vi "SEN_Loop.vi"() -> ()   [LabVIEW 2023, in "Swerve_Odometry_SEN.lvlib"]
uses:
  Swerve_Odometry_SEN.lvlib
  RoboRIO Utilities/Global_STOP.vi
  ENUM_SEN_Action.ctl
  ENUM_SEN_State.ctl
  Global_SEN_Data Out.vi
  Global_CMD_SEN_Data In.vi
  Cluster_TRANSLATION2D.ctl
  Cluster_ROTATION2D.ctl
  Cluster_POSE2D.ctl
  Cluster_SWERVE_DRIVE_MODULE_POSITION.ctl
  Cluster_SWERVE_DRIVE_ODOMETRY.ctl
  SwerveDrive/Global_ACT_Data Out.vi
  PigeonIMU/Global_SEN_Data Out.vi
panel:
  out "SWERVE_DRIVE_ODOMETRY":T1={"POSE"={"TRANSLATION"={"X"=0.0, "Y"=0.0}, "ROTATION"={"VALUE"=0.0, "COS"=1.0, "SIN"=0.0}}, "GyroOffset"={"VALUE"=0.0, "COS"=1.0, "SIN"=0.0}, "PreviousAngle"={"VALUE"=0.0, "COS"=1.0, "SIN"=0.0}, "PrevTime"=0.0, "PrevModulePosition"=[], "NumModules"=0} {"PrevModulePosition"."Angle"."SIN" format="%13.4f"; "PrevModulePosition"."Angle"."COS" format="%13.4f"; "PrevModulePosition"."Angle"."VALUE" format="%13.4f"; "PreviousAngle"."SIN" format="%13.4f"; "PreviousAngle"."COS" format="%13.4f"; "PreviousAngle"."VALUE" format="%13.4f"; "GyroOffset"."SIN" format="%13.4f"; "GyroOffset"."COS" format="%13.4f"; "GyroOffset"."VALUE" format="%13.4f"; "POSE"."ROTATION"."SIN" format="%13.4f"; "POSE"."ROTATION"."COS" format="%13.4f"; "POSE"."ROTATION"."VALUE" format="%13.4f"; "POSE"."TRANSLATION"."Y" format="%14.3f"; "POSE"."TRANSLATION"."X" format="%14.3f"}
  out "Is Tracking":bool
  out "Cycle Time (S)":dbl format="%.3g"
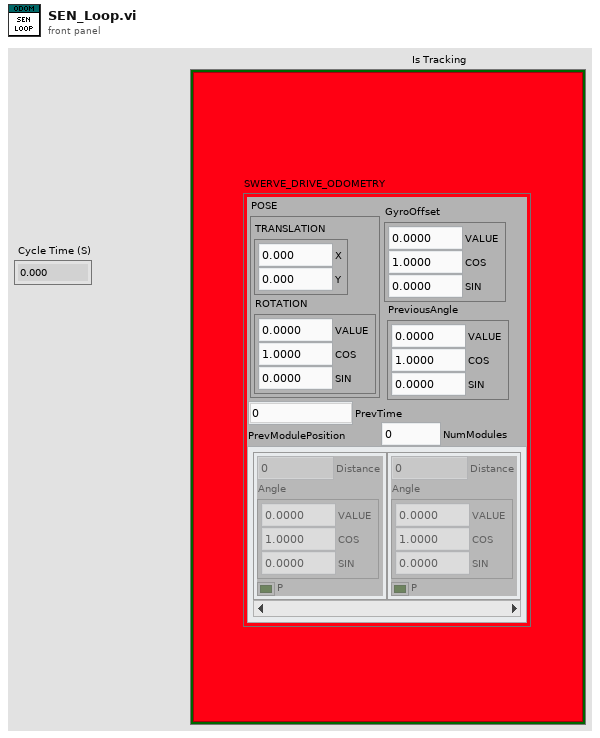
[diagram p1: front panel]
types:
  T1 = typedef "Swerve_Odometry_SEN.lvlib/Cluster_SWERVE_DRIVE_ODOMETRY.ctl" = cluster{"POSE":T2, "GyroOffset":T4, "PreviousAngle":T4, "PrevTime":dbl, "PrevModulePosition":T5[], "NumModules":i32}
  T2 = typedef "Swerve_Odometry_SEN.lvlib/Cluster_POSE2D.ctl" = cluster{"TRANSLATION":T3, "ROTATION":T4}
  T3 = typedef "Swerve_Odometry_SEN.lvlib/Cluster_TRANSLATION2D.ctl" = cluster{"X":dbl, "Y":dbl}
  T4 = typedef "Swerve_Odometry_SEN.lvlib/Cluster_ROTATION2D.ctl" = cluster{"VALUE":dbl, "COS":dbl, "SIN":dbl}
  T5 = typedef "Swerve_Odometry_SEN.lvlib/Cluster_SWERVE_DRIVE_MODULE_POSITION.ctl" = cluster{"Distance":dbl, "Angle":T4, "P":bool}
  T6 = typedef "Swerve_Odometry_SEN.lvlib/ENUM_SEN_State.ctl" = enum16{"Startup", "Reset", "Enable", "Tracking", "Disable", "Shutdown"}
  T7 = typedef "Swerve_Odometry_SEN.lvlib/ENUM_SEN_Action.ctl" = enum16{"No Action", "Reset Time", "Reset Enable", "Reset Disable", "Read Enable", "Read Disable", "Update Module Positions", "Update Rotation", "Create New Odometry", "Update Odometry"}
  T8 = typedef "Swerve_Odometry_SEN.lvlib/Cluster_SWERVE_DRIVE_KINEMATICS.ctl" = cluster{"NumModules":i32, "InverseKinematics":T9, "ForwardKinematics":T9, "Modules":T3[], "PrevCoR":T3, "SavedModuleStates":T10[]}
  T9 = typedef "NI_Matrix.lvlib/RealMatrix.ctl" = dbl[][]
  T10 = typedef "Swerve_Odometry_SEN.lvlib/Cluster_SWERVE_DRIVE_MODULE_STATE.ctl" = cluster{"Speed":dbl, "Angle":T4}
  T11 = cluster{"State":T6, "Previous State":T6, "Current Time":timestamp, "Previous Time":timestamp, "Start Time":timestamp, "Target Time (ms)":u32, "Cycle Time(S)":dbl, "Tracking":bool, "Offset Values":cluster{"Y":dbl, "X":dbl, "Degrees":dbl}, "Module Positions":T5[], "SWERVE_DRIVE_ODOMETRY":T1, "robot POSE":T2, "Pigeon ROTATION":T4, "SWERVE_DRIVE_KINEMATICS Out":T8}
  T12 = typedef "Cluster_Yaw Pitch Roll in Deg.ctl" = cluster{"Yaw":dbl, "Pitch":dbl, "Roll":dbl}
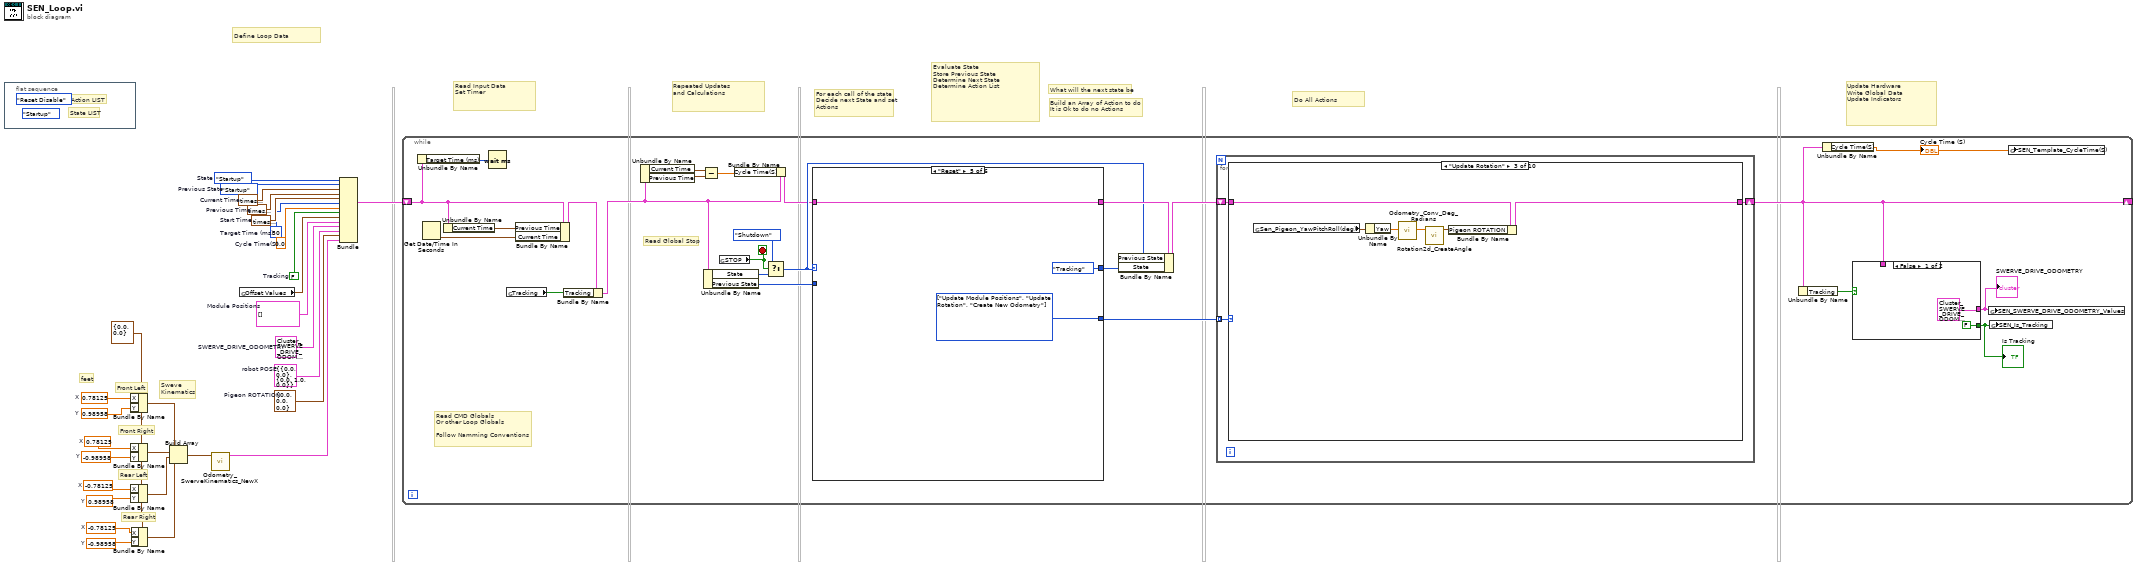
[diagram p0: block diagram]
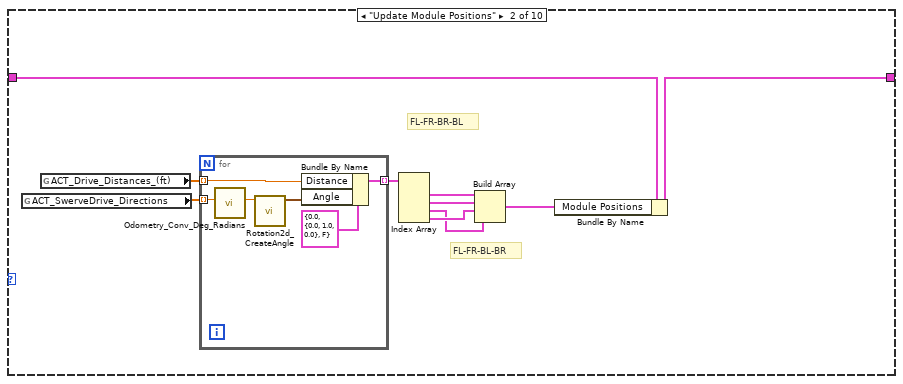
[diagram p3: hidden frame]
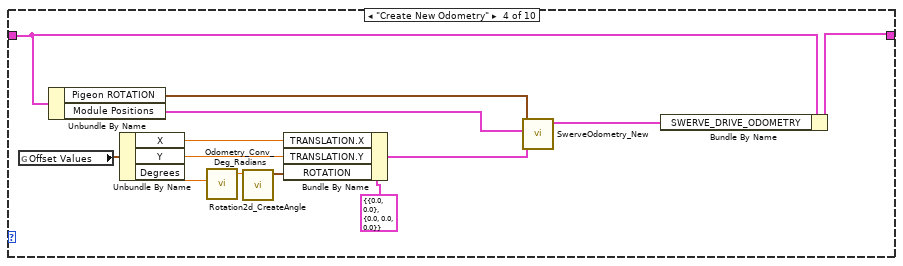
[diagram p4: hidden frame]
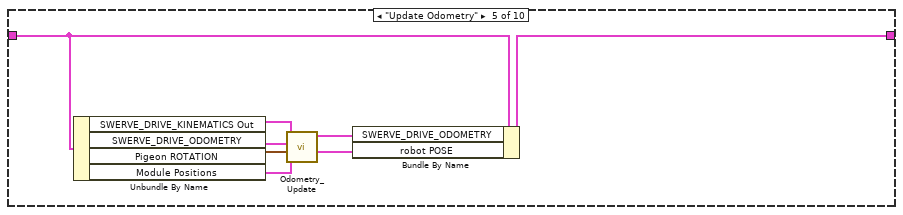
[diagram p5: hidden frame]
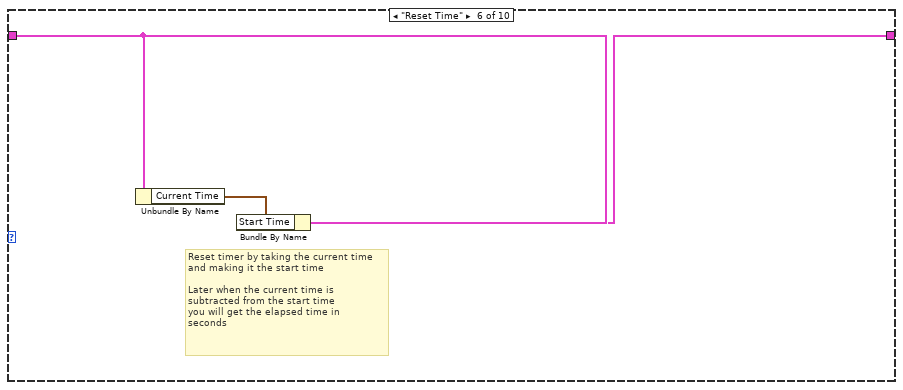
[diagram p6: hidden frame]
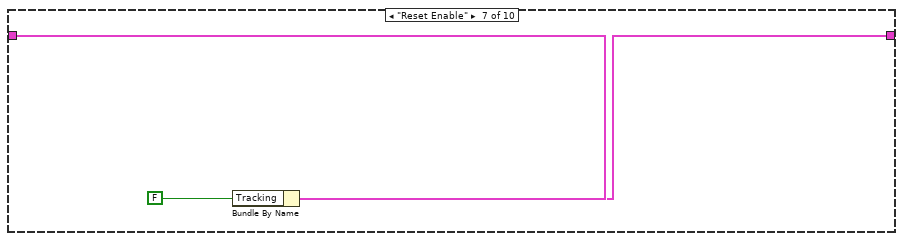
[diagram p7: hidden frame]
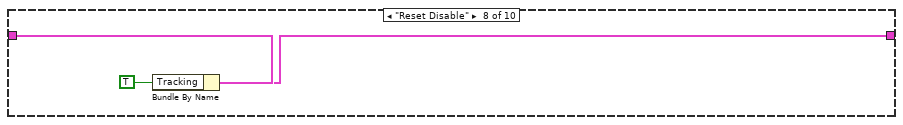
[diagram p8: hidden frame]
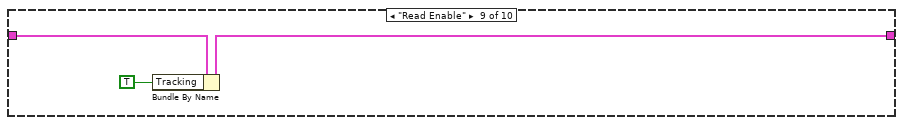
[diagram p9: hidden frame]
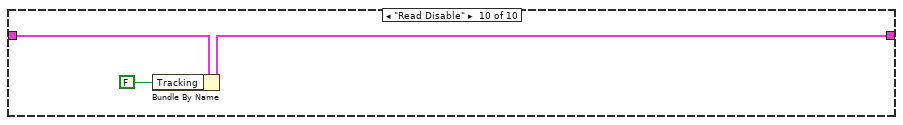
[diagram p10: hidden frame]
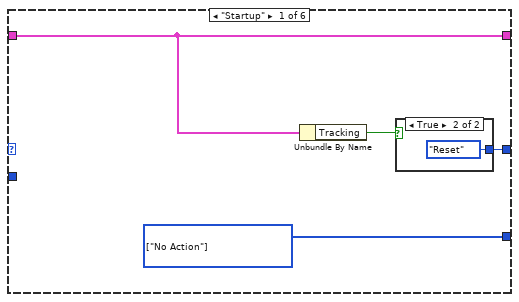
[diagram p11: hidden frame]
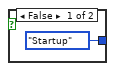
[diagram p12: hidden frame]
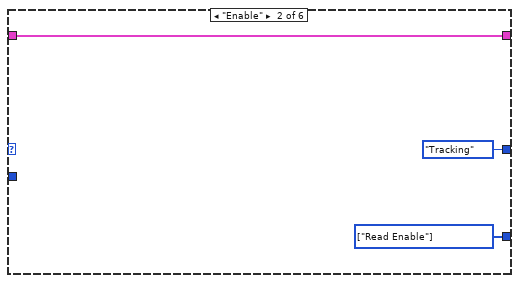
[diagram p13: hidden frame]
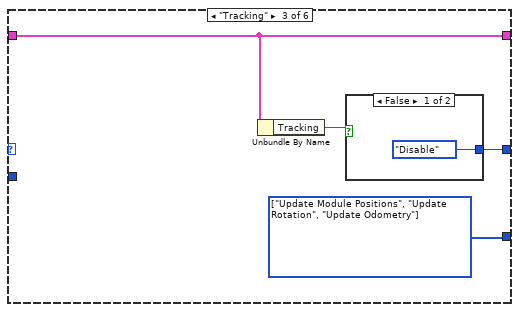
[diagram p14: hidden frame]
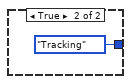
[diagram p15: hidden frame]
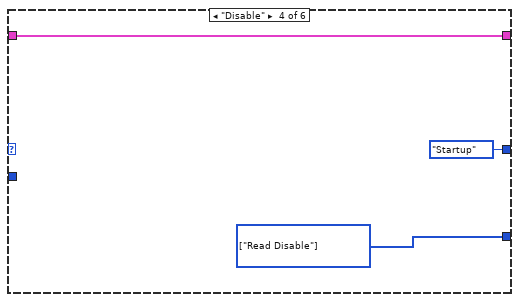
[diagram p16: hidden frame]
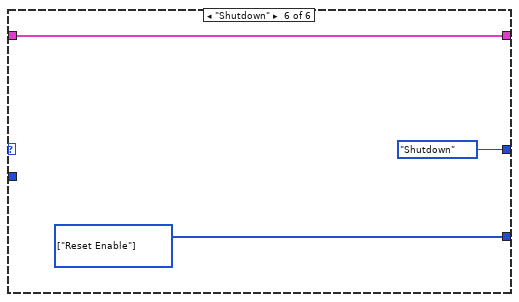
[diagram p17: hidden frame]
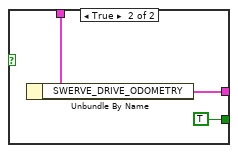
[diagram p18: hidden frame]
diagram:
  w9 = T3 {"X"=0.0, "Y"=0.0} ("TRANSLATION")
  w8 = -0.78125  # X
  w7 = -0.98958  # Y
  w11 = -0.78125  # X
  w10 = 0.98958  # Y
  w13 = 0.78125  # X
  w12 = -0.98958  # Y
  w15 = 0.78125  # X
  w14 = 0.98958  # Y
  w17 = T4 {"VALUE"=0.0, "COS"=0.0, "SIN"=0.0}  # Pigeon ROTATION
  w18 = T2 {"TRANSLATION"={"X"=0.0, "Y"=0.0}, "ROTATION"={"VALUE"=0.0, "COS"=1.0, "SIN"=0.0}}  # robot POSE
  w16 = T1 {"POSE"={"TRANSLATION"={"X"=0.0, "Y"=0.0}, "ROTATION"={"VALUE"=0.0, "COS"=1.0, "SIN"=0.0}}, "GyroOffset"={"VALUE"=0.0, "COS"=1.0, "SIN"=0.0}, "PreviousAngle"={"VALUE"=0.0, "COS"=1.0, "SIN"=0.0}, "PrevTime"=0.0, "PrevModulePosition"=[], "NumModules"=0}  # SWERVE_DRIVE_ODOMETRY
  w19 = T5[] []  # Module Positions
  w21 = FALSE  # Tracking
  w23 = 0.0  # Cycle Time(S)
  w24 = ENUM_SEN_State."Startup"  # Previous State
  w25 = timestamp(0 s since 1904-01-01)  # Previous Time
  w26 = u32 50  # Target Time (ms)
  w27 = timestamp(0 s since 1904-01-01)  # Start Time
  w28 = timestamp(0 s since 1904-01-01)  # Current Time
  w29 = ENUM_SEN_State."Startup"  # State
  # "feet"
  # "Sweve\nKinematics"
  # "Rear Right"
  # "Rear Left"
  # "Front Right"
  # "Front Left"
  # "Build an Array of Action to do\nIt is Ok to do no Actions"
  # "What will the next state be"
  # "For each call of the state\nDecide next State and set\nActions"
  # "Define Loop Data"
  # "Repeated Updates\nand Calculations"
  # "Read Input Data\nSet Timer"
  # "Evaluate State\nStore Previous State\nDetermine Next State\nDetermine Action List"
  # "Do All Actions"
  # "Update Hardware\nWrite Global Data\nUpdate Indicators"
  n1 = flat-sequence {
    frame #0 {
      (unwired) ENUM_SEN_State."Startup" ("State")
      (unwired) ENUM_SEN_Action."Reset Disable" ("Action")
      # "State LIST"
      # "Action LIST"
    }
  }
  n2 = Bundle By Name(cluster=w9, "X"=w15, "Y"=w14) -> (w5:T3)
  n3 = Bundle By Name(cluster=w9, "X"=w13, "Y"=w12) -> (w4:T3)
  n4 = Bundle By Name(cluster=w9, "X"=w11, "Y"=w10) -> (w3:T3)
  n5 = Bundle By Name(cluster=w9, "X"=w8, "Y"=w7) -> (w2:T3)
  n6 = Build Array(w5, w4, w3, w2) -> (w1:T3[])
  n7 = call "Odometry_SwerveKinematics_NewX.vi"("Distances From Center"=w1) -> ("SWERVE_DRIVE_KINEMATICS Out"=w6:T8)  [unwired: 10 in]
  n8 = global read "Global_CMD_SEN_Data In.vi" "Offset Values"() -> (w20:cluster{"Y":dbl, "X":dbl, "Degrees":dbl})
  n9 = Bundle("State"=w29, "Previous State"=w24, "Current Time"=w28, "Previous Time"=w25, "Start Time"=w27, "Target Time (ms)"=w26, "Cycle Time(S)"=w23, "Tracking"=w21, "Offset Values"=w20, "Module Positions"=w19, "SWERVE_DRIVE_ODOMETRY"=w16, "robot POSE"=w18, "Pigeon ROTATION"=w17, "SWERVE_DRIVE_KINEMATICS Out"=w6) -> (w22:T11)  [unwired: 1 in]
  n10 = while {
    shift-right: [w31] -> _
    shift-left: w22 -> [w45]
    stop <- w50 stop-if-true
    # "Read CMD Globals\nOr other Loop Globals\n\nFollow Namming Conventions"
    # "Read Global Stop"
    n11 = Unbundle By Name(w45) -> ("Target Time (ms)"=w47:u32)
    n12 = Get Date/Time In Seconds() -> (seconds since 1Jan1904=w54:timestamp)
    n13 = Unbundle By Name(w45) -> ("Current Time"=w46:timestamp)
    n14 = Wait (ms)(milliseconds to wait=w47) -> ()  [unwired: 1 out]
    n15 = global read "Global_CMD_SEN_Data In.vi" "Tracking"() -> (w33:bool)
    n16 = Bundle By Name(cluster=w45, "Previous Time"=w46, "Current Time"=w54) -> (w35:T11)
    n17 = Bundle By Name(cluster=w35, "Tracking"=w33) -> (w34:T11)
    n18 = Unbundle By Name(w34) -> ("Current Time"=w41:timestamp, "Previous Time"=w42:timestamp)
    n19 = Subtract(x=w41, y=w42) -> (x-y=w39:dbl)
    n20 = Unbundle By Name(w34) -> ("State"=w48:T6, "Previous State"=w44:T6)
    n21 = global read "Global_STOP.vi" "STOP"() -> (w50:bool)
    n22 = Bundle By Name(cluster=w34, "Cycle Time(S)"=w39) -> (w40:T11)
    n23 = Select(t=ENUM_SEN_State."Shutdown" ("State"), s=w50, f=w48) -> (s? t:f=w43:T6)
    n24 = case shown="\"Reset\"" w43 {
      tunnel: w40 -> [w118 w125 w126 w134 w137 w140]
      tunnel: [w118 w125 w126 w134 w137 w140] -> w52
      tunnel: [w119 ENUM_SEN_State."Tracking" ("State") w129 ENUM_SEN_State."Startup" ("State") ENUM_SEN_State."Tracking" ("State") ENUM_SEN_State."Shutdown" ("State")] -> w51
      tunnel: [w120 w123 w128 w132 w135 w138] -> w38
      tunnel: w44 -> [_ _ _ _ _ _]
      frame "Startup" {
        w120 = T7[] [enum."No Action"] items=["No Action", "Reset Time", "Reset Enable", "Reset Disable", "Read Enable", "Read Disable", "Update Module Positions", "Update Rotation", "Create New Odometry", "Update Odometry"] ("Actions")
        n25 = Unbundle By Name(w118) -> ("Tracking"=w117:bool)
        n26 = case shown="True" w117 {
          tunnel: [ENUM_SEN_State."Startup" ("State") ENUM_SEN_State."Reset" ("State")] -> w119
          frame False {
          }
          frame True {
          }
        }
      }
      frame "Enable" {
        w123 = T7[] [enum."Read Enable"] items=["No Action", "Reset Time", "Reset Enable", "Reset Disable", "Read Enable", "Read Disable", "Update Module Positions", "Update Rotation", "Create New Odometry", "Update Odometry"] ("Actions")
      }
      frame "Tracking" {
        w128 = T7[] [enum."Update Module Positions", enum."Update Rotation", enum."Update Odometry"] items=["No Action", "Reset Time", "Reset Enable", "Reset Disable", "Read Enable", "Read Disable", "Update Module Positions", "Update Rotation", "Create New Odometry", "Update Odometry"] ("Actions")
        n27 = Unbundle By Name(w126) -> ("Tracking"=w127:bool)
        n28 = case shown="False" w127 {
          tunnel: [ENUM_SEN_State."Disable" ("State") ENUM_SEN_State."Tracking" ("State")] -> w129
          frame False {
          }
          frame True {
          }
        }
      }
      frame "Disable" {
        w132 = T7[] [enum."Read Disable"] items=["No Action", "Reset Time", "Reset Enable", "Reset Disable", "Read Enable", "Read Disable", "Update Module Positions", "Update Rotation", "Create New Odometry", "Update Odometry"] ("Actions")
      }
      frame "Reset" {
        w135 = T7[] [enum."Update Module Positions", enum."Update Rotation", enum."Create New Odometry"] items=["No Action", "Reset Time", "Reset Enable", "Reset Disable", "Read Enable", "Read Disable", "Update Module Positions", "Update Rotation", "Create New Odometry", "Update Odometry"] ("Actions")
      }
      frame "Shutdown" {
        w138 = T7[] [enum."Reset Enable"] items=["No Action", "Reset Time", "Reset Enable", "Reset Disable", "Read Enable", "Read Disable", "Update Module Positions", "Update Rotation", "Create New Odometry", "Update Odometry"] ("Actions")
      }
    }
    n29 = Bundle By Name(cluster=w52, "Previous State"=w43, "State"=w51) -> (w53:T11)
    n30 = for {
      tunnel: w38 -> [w57] mode=indexing
      shift-right: [w56] -> w31
      shift-left: w53 -> [w55]
      n31 = case shown="\"Update Rotation\"" w57 {
        tunnel: w55 -> [w58 w61 w79 w91 w97 w104 w107 w110 w113 w116]
        tunnel: [w58 w60 w78 w89 w96 w103 w106 w109 w112 w115] -> w56
        frame "No Action" {
        }
        frame "Update Module Positions" {
          # "FL-FR-BR-BL"
          # "FL-FR-BL-BR"
          n32 = global read "Global_ACT_Data Out.vi" "ACT_SwerveDrive_Directions"() -> (w67:dbl[])
          n33 = global read "Global_ACT_Data Out.vi" "ACT_Drive_Distances_(ft)"() -> (w68:dbl[])
          n34 = for {
            tunnel: w68 -> [w73] mode=indexing
            tunnel: w67 -> [w70] mode=indexing
            tunnel: [w72] -> w66 mode=indexing
            n35 = call "Odometry_Conv_Deg_Radians.vi"("Degress"=w70) -> ("Radians"=w71:dbl)  [unwired: 10 in]
            n36 = call "Rotation2d_CreateAngle.vi"("Angle (Radians)"=w71) -> ("ROTATION"=w69:T4)  [unwired: 10 in]
            n37 = Bundle By Name(cluster=T5 {"Distance"=0.0, "Angle"={"VALUE"=0.0, "COS"=1.0, "SIN"=0.0}, "P"=FALSE} ("SWERVE_DRIVE_MODULE_POSITION"), "Distance"=w73, "Angle"=w69) -> (w72:T5)
          }
          n38 = Index Array(array=w66) -> (element #1=w65:T5, element #2=w64:T5, element #3=w62:T5, element #4=w63:T5)  [unwired: 4 in]
          n39 = Build Array(w65, w64, w63, w62) -> (w59:T5[])
          n40 = Bundle By Name(cluster=w61, "Module Positions"=w59) -> (w60:T11)
        }
        frame "Update Rotation" {
          n41 = global read "Global_SEN_Data Out.vi" "Sen_Pigeon_YawPitchRoll(deg)"() -> (w80:T12)
          n42 = Unbundle By Name(w80) -> ("Yaw"=w76:dbl)
          n43 = call "Odometry_Conv_Deg_Radians.vi"("Degress"=w76) -> ("Radians"=w75:dbl)  [unwired: 10 in]
          n44 = call "Rotation2d_CreateAngle.vi"("Angle (Radians)"=w75) -> ("ROTATION"=w77:T4)  [unwired: 10 in]
          n45 = Bundle By Name(cluster=w79, "Pigeon ROTATION"=w77) -> (w78:T11)
        }
        frame "Create New Odometry" {
          n46 = global read "Global_CMD_SEN_Data In.vi" "Offset Values"() -> (w93:cluster{"Y":dbl, "X":dbl, "Degrees":dbl})
          n47 = Unbundle By Name(w91) -> ("Pigeon ROTATION"=w88:T4, "Module Positions"=w92:T5[])
          n48 = Unbundle By Name(w93) -> ("X"=w81:dbl, "Y"=w82:dbl, "Degrees"=w87:dbl)
          n49 = call "Odometry_Conv_Deg_Radians.vi"("Degress"=w87) -> ("Radians"=w83:dbl)  [unwired: 10 in]
          n50 = call "Rotation2d_CreateAngle.vi"("Angle (Radians)"=w83) -> ("ROTATION"=w85:T4)  [unwired: 10 in]
          n51 = Bundle By Name(cluster=T2 {"TRANSLATION"={"X"=0.0, "Y"=0.0}, "ROTATION"={"VALUE"=0.0, "COS"=0.0, "SIN"=0.0}} ("sumPOSE"), "TRANSLATION.X"=w81, "TRANSLATION.Y"=w82, "ROTATION"=w85) -> (w84:T2)
          n52 = call "SwerveOdometry_New.vi"("InitialPose"=w84, "Module Positions"=w92, "GyroAngle"=w88) -> ("SWERVE_DRIVE_ODOMETRY Out"=w90:T1)  [unwired: 8 in]
          n53 = Bundle By Name(cluster=w91, "SWERVE_DRIVE_ODOMETRY"=w90) -> (w89:T11)
        }
        frame "Update Odometry" {
          n54 = Unbundle By Name(w97) -> ("SWERVE_DRIVE_KINEMATICS Out"=w101:T8, "SWERVE_DRIVE_ODOMETRY"=w100:T1, "Pigeon ROTATION"=w99:T4, "Module Positions"=w98:T5[])
          n55 = call "Odometry_Update.vi"("Module Positions"=w98, "GyroAngle"=w99, "In SWERVE_DRIVE_ODOMETRY"=w100, "SWERVE_DRIVE_KINEMATICS"=w101) -> ("Robot POSE Out"=w95:T2, "Out SWERVE_DRIVE_ODOMETRY Out"=w94:T1)  [unwired: 5 in, 1 out]
          n56 = Bundle By Name(cluster=w97, "SWERVE_DRIVE_ODOMETRY"=w94, "robot POSE"=w95) -> (w96:T11)
        }
        frame "Reset Time" {
          # "Reset timer by taking the current time\nand making it the start time\n\nLater when the current time is \nsubtracted from the start time\nyou will get the elapsed time in \nseconds"
          n57 = Unbundle By Name(w104) -> ("Current Time"=w102:timestamp)
          n58 = Bundle By Name(cluster=w104, "Start Time"=w102) -> (w103:T11)
        }
        frame "Reset Enable" {
          n59 = Bundle By Name(cluster=w107, "Tracking"=FALSE ("Read Enable")) -> (w106:T11)
        }
        frame "Reset Disable" {
          n60 = Bundle By Name(cluster=w110, "Tracking"=TRUE ("Read Enable")) -> (w109:T11)
        }
        frame "Read Enable" {
          n61 = Bundle By Name(cluster=w113, "Tracking"=TRUE ("Read Enable")) -> (w112:T11)
        }
        frame "Read Disable" {
          n62 = Bundle By Name(cluster=w116, "Tracking"=FALSE ("Read Enable")) -> (w115:T11)
        }
      }
    }
    n63 = Unbundle By Name(w31) -> ("Tracking"=w36:bool)
    n64 = Unbundle By Name(w31) -> ("Cycle Time(S)"=w37:dbl)
    "Cycle Time (S)" <- w37
    n65 = case shown="False" w36 {
      tunnel: w31 -> [_ w145]
      tunnel: [T1 {"POSE"={"TRANSLATION"={"X"=0.0, "Y"=0.0}, "ROTATION"={"VALUE"=0.0, "COS"=1.0, "SIN"=0.0}}, "GyroOffset"={"VALUE"=0.0, "COS"=1.0, "SIN"=0.0}, "PreviousAngle"={"VALUE"=0.0, "COS"=1.0, "SIN"=0.0}, "PrevTime"=0.0, "PrevModulePosition"=[], "NumModules"=0} ("SWERVE_DRIVE_ODOMETRY") w144] -> w30
      tunnel: [FALSE TRUE] -> w32
      frame False {
      }
      frame True {
        n66 = Unbundle By Name(w145) -> ("SWERVE_DRIVE_ODOMETRY"=w144:T1)
      }
    }
    "Is Tracking" <- w32
    "SWERVE_DRIVE_ODOMETRY" <- w30
    n67 = global write "Global_SEN_Data Out.vi" "SEN_SWERVE_DRIVE_ODOMETRY_Values"(w30) -> ()
    n68 = global write "Global_SEN_Data Out.vi" "SEN_Is_Tracking"(w32) -> ()
    n69 = global write "Global_SEN_Data Out.vi" "SEN_Template_CycleTime(S)"(w37) -> ()
  }
